vi "Flush Entries.vi"(8 "error in (no error)":errorcluster, 11 "CLILogger in":refnum<class "CLILogger.lvclass">) -> (0 "error out":errorcluster, 2 "Entries":T1[](array[typedef]), 3 "CLILogger out":refnum<class "CLILogger.lvclass">)   [LabVIEW 2020, in "GPackTools.lvlib" / "CLILogger.lvclass"]
uses:
  CLILogger.lvclass
  Log Entry.ctl
  CLILogger.lvclass/CLILogger.ctl
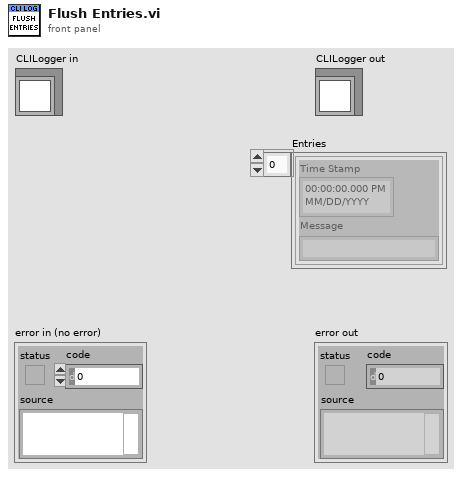
[diagram p1: front panel]
types:
  T1 = typedef "GPackTools.lvlib/CLILogger.lvclass/Log Entry.ctl" = cluster{"Time Stamp":timestamp, "Message":string}
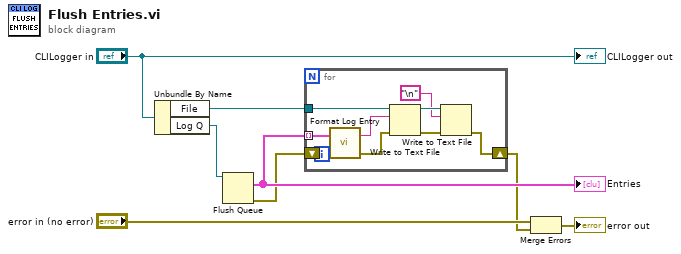
[diagram p0: block diagram]
diagram:
  n1 = Unbundle By Name("CLILogger in") -> ("File"=w4:refnum<file>, "Log Q"=w6:refnum<queue>)
  n2 = Flush Queue(queue=w6) -> (remaining elements=w3:T1[], error out=w2:errorcluster)  [unwired: 1 in, 1 out]
  "Entries" <- w3
  n3 = for {
    tunnel: w4 -> [w15]
    tunnel: w3 -> [w16] mode=indexing
    shift-right: [w9] -> w1
    shift-left: w2 -> [w10]
    n4 = call "Format Log Entry.vi"("Log Entry"=w16) -> ("Entry String"=w14:string)  [unwired: 2 in]
    n5 = Write to Text File(file (use dialog)=w15, text=w14, error in=w10) -> (refnum out=w13:refnum<file>, error out=w11:errorcluster)  [unwired: 1 in, 1 out]
    n6 = Write to Text File(file (use dialog)=w13, text="\n", error in=w11) -> (error out=w9:errorcluster)  [unwired: 1 in, 2 out]
  }
  n7 = Merge Errors("error in (no error)", w1) -> (→"error out":errorcluster)
  "CLILogger out" <- "CLILogger in"
